vi "Save Data I16.vi"(8 "error in (no error)":errorcluster, 9 "I32 data":i32[][](array[numeric]), 10 "I16 data":i16[][](array[numeric]), 11 "Pulse Driver in":refnum<class "Pulse Driver.lvclass">) -> (0 "error out":errorcluster, 3 "Pulse Driver out":refnum<class "Pulse Driver.lvclass">)   [LabVIEW 2016, in "Pulse Driver.lvclass"]
uses:
  Pulse Driver.lvclass
  C:/github/NHMFL_Core/Libraries/Instruments/Instrument Driver/Instrument Driver.lvclass
  Pulse Driver.lvclass/Pulse Driver.ctl
  Instrument Driver/Instrument Driver.lvclass/Instrument Driver.ctl
  Read tdms file.vi
  Instrument Driver/Read Group name.vi
  Instrument Driver/Read Channel names.vi
  Read Binary sample width.vi
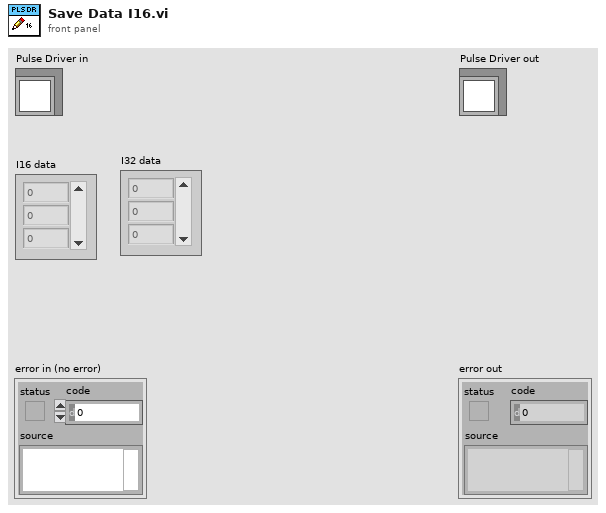
[diagram p1: front panel]
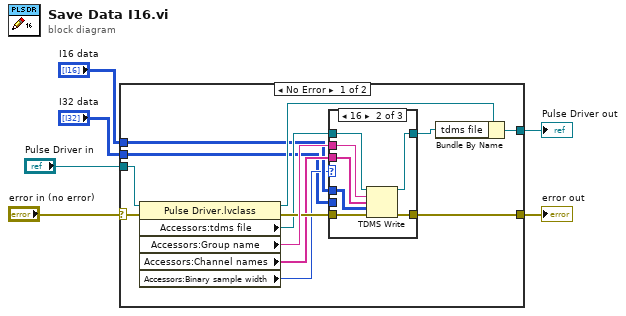
[diagram p0: block diagram]
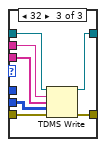
[diagram p3: hidden frame]
diagram:
  n1 = case shown="No Error" "error in (no error)" {
    selector: "error in (no error)" -> [w9 w37]
    tunnel: [w10 w37] -> w5
    tunnel: [w11 w36] -> w3
    tunnel: "Pulse Driver in" -> [w12 w36]
    tunnel: "I16 data" -> [w13 _]
    tunnel: "I32 data" -> [w7 _]
    frame No Error {
      n2 = property class="Pulse Driver.lvclass"(reference=w12, error in=w9) -> (reference out=w15:refnum<class "Pulse Driver.lvclass">, error out=w18:errorcluster, "Accessors:tdms file"=w16:refnum<k34>, "Accessors:Group name"=w19:string, "Accessors:Channel names"=w17:string[], "Accessors:Binary sample width"=w8:i32)
      n3 = case shown="16" w8 {
        tunnel: w19 -> [_ w28 w35]
        tunnel: w18 -> [w21 w27 w34]
        tunnel: w17 -> [_ w26 w33]
        tunnel: w16 -> [w20 w25 w32]
        tunnel: [w20 w24 w31] -> w14
        tunnel: w13 -> [_ w23 _]
        tunnel: [w21 w22 w30] -> w10
        tunnel: w7 -> [_ _ w29]
        frame 0, Default {
        }
        frame 16 {
          n4 = TDMS Write(0:w25, 5:w28, 7:w26, 9:w23, 11:w27) -> (4:w24:refnum<k34>, 15:w22:errorcluster)  [unwired: 1 in, 2 out]
        }
        frame 32 {
          n5 = TDMS Write(0:w32, 5:w35, 7:w33, 9:w29, 11:w34) -> (4:w31:refnum<k34>, 15:w30:errorcluster)  [unwired: 1 in, 2 out]
        }
      }
      n6 = Bundle By Name(cluster=w15, "tdms file"=w14) -> (w11:refnum<class "Pulse Driver.lvclass">)
    }
    frame Error {
    }
  }
  "error out" <- w5
  "Pulse Driver out" <- w3
